vi "display lines.vi"(8 "error in (no error)":errorcluster, 11 "USB-6000 in":refnum<class "USB-6000.lvclass">) -> (0 "error out":errorcluster, 1 "Values":i32[](array[numeric]), 2 "Lines":string[](array[string]), 3 "USB-6000 out":refnum<class "USB-6000.lvclass">)   [LabVIEW 2025, in "USB IO.lvlib" / "USB-6000.lvclass"]
uses:
  USB-6000.lvclass
  USB-6000.lvclass/USB-6000.ctl
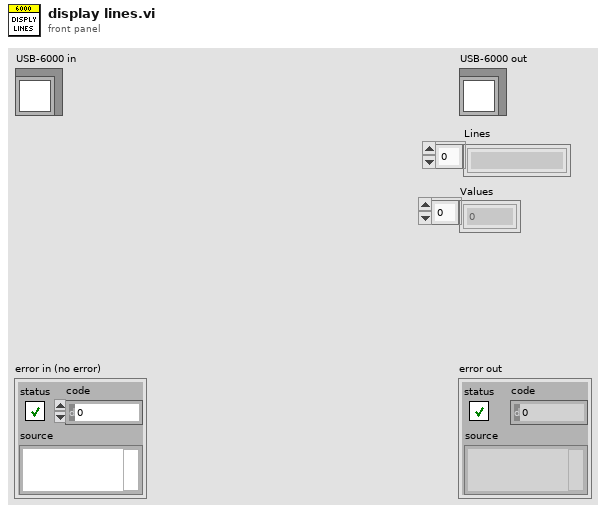
[diagram p1: front panel]
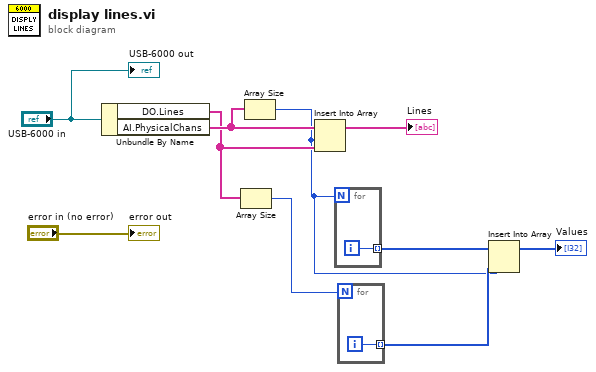
[diagram p0: block diagram]
diagram:
  n1 = Unbundle By Name("USB-6000 in") -> ("DO.Lines"=w8:tag[], "AI.PhysicalChans"=w10:tag[])
  n2 = Array Size(array=w8) -> (size(s)=w7:i32)
  n3 = Array Size(array=w10) -> (size(s)=w4:i32)
  n4 = Insert Into Array(array=w10, index=w4, new element=w8) -> (→"Lines":tag[])
  n5 = for {
    N: w4 -> [_]
    tunnel: [w11] -> w6 mode=indexing
    i -> [w11]
  }
  n6 = for {
    N: w7 -> [_]
    tunnel: [w12] -> w5 mode=indexing
    i -> [w12]
  }
  n7 = Insert Into Array(array=w6, index=w4, new element=w5) -> (→"Values":i32[])
  "error out" <- "error in (no error)"
  "USB-6000 out" <- "USB-6000 in"
